vi "Classify.vi"(4 "Python Directory Path":path=path "", 5 "input cluster":T1, 6 "Ref_filepath":path=path "../src/deterministic_classifier/refs/Si(111)-cornerhole.npy" caption="filename", 7 "Filename_1":path) -> (0 "CCR":string, 1 "Good Image":bool, 2 "Tip Change?":bool, 3 "FRC":string)   [LabVIEW 2025]
panel:
  out "result string":string
  out "standard output":string
  out "standard error":string
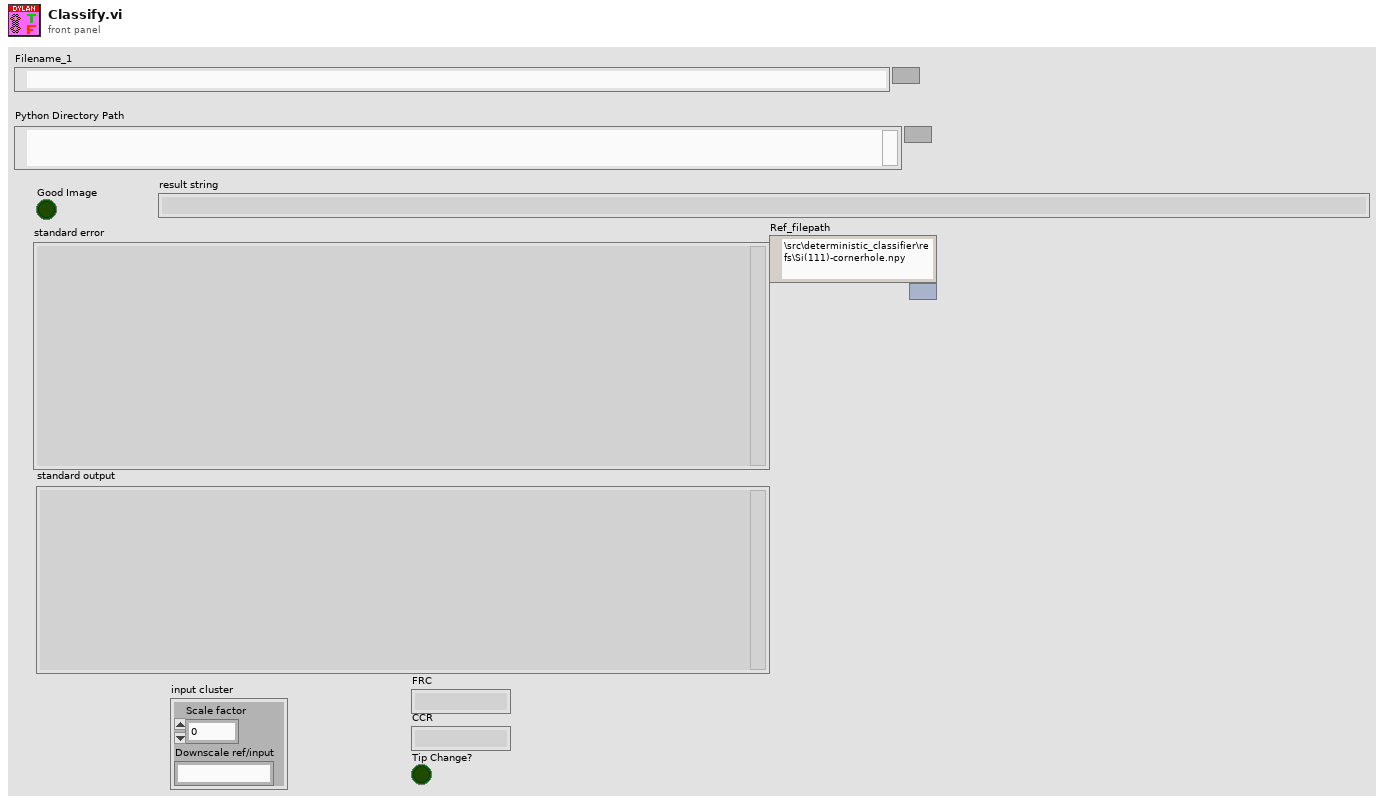
[diagram p1: front panel]
types:
  T1 = cluster{"Scale factor":sgl, "Downscale ref/input":string}
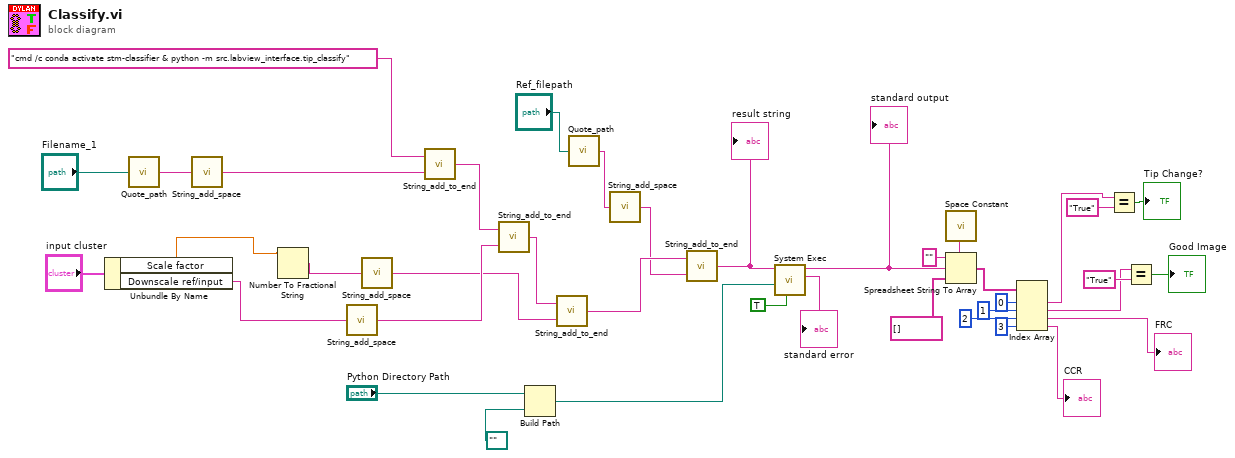
[diagram p0: block diagram]
diagram:
  n1 = Unbundle By Name("input cluster") -> ("Scale factor"=w25:sgl, "Downscale ref/input"=w30:string)
  n2 = call "Quote_path.vi"("File path in"="Filename_1") -> ("result string"=w36:string)
  n3 = call "String_add_space.vi"("result string in"=w36) -> ("result string out"=w35:string)
  n4 = Number To Fractional String(number=w25) -> (F-format string=w24:string)  [unwired: 3 in]
  n5 = call "String_add_space.vi"("result string in"=w30) -> ("result string out"=w27:string)
  n6 = call "String_add_space.vi"("result string in"=w24) -> ("result string out"=w26:string)
  n7 = call "String_add_to_end.vi"("Addition String"=w35, "command line"="cmd /c conda activate stm-classifier & python -m src.labview_interface.tip_classify") -> ("result string"=w29:string)
  n8 = call "String_add_to_end.vi"("Addition String"=w27, "command line"=w29) -> ("result string"=w28:string)
  n9 = Build Path(base path="Python Directory Path", name or relative path=path "..") -> (appended path=w6:path)
  n10 = call "String_add_to_end.vi"("Addition String"=w26, "command line"=w28) -> ("result string"=w3:string)
  n11 = call "Quote_path.vi"("File path in"="Ref_filepath") -> ("result string"=w4:string)
  n12 = call "String_add_space.vi"("result string in"=w4) -> ("result string out"=w2:string)
  n13 = call "String_add_to_end.vi"("Addition String"=w2, "command line"=w3) -> ("result string"=w1:string)
  "result string" <- w1
  n14 = call <vilib>:"System Exec.vi"("run minimized? (F)"=TRUE, "working directory"=w6, "command line"=w1) -> ("standard error"=→"standard error":string, "standard output"=w23:string)  [unwired: 5 in, 2 out]
  "standard output" <- w23
  n15 = call <vilib>:"Space Constant.vi"() -> ("String"=w22:string)
  n16 = Spreadsheet String To Array(delimiter (Tab)=w22, format string="", spreadsheet string=w23, array type (2D Dbl)=string[] []) -> (array=w19:string[])
  n17 = Index Array(array=w19, index #1=0 ("index"), index #2=1 ("index"), index #3=2 ("index"), index #4=3 ("index")) -> (element #1=w9:string, element #2=w12:string, element #3=→"FRC":string, element #4=→"CCR":string)
  n18 = Equal?(x=w9, y="True") -> (x = y?=→"Tip Change?":bool)
  n19 = Equal?(x=w12, y="True") -> (x = y?=→"Good Image":bool)
